vi "ConvertDMDTypeToHumanReadable.vi"(11 "UserVarPtr in":i32) -> (3 "String":string)   [LabVIEW 2013, in "alpD41.lvlib"]
uses:
  alpD41.lvlib
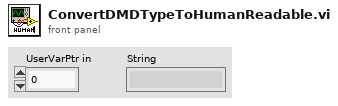
[diagram p1: front panel]
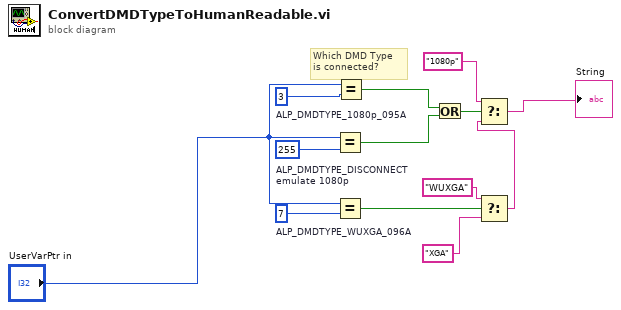
[diagram p0: block diagram]
diagram:
  w5 = u32 7  # ALP_DMDTYPE_WUXGA_096A
  w1 = u32 255  # ALP_DMDTYPE_DISCONNECT emulate 1080p
  w2 = u32 3  # ALP_DMDTYPE_1080p_095A
  # "Which DMD Type\nis connected?"
  n1 = Equal?(x="UserVarPtr in", y=w1) -> (x = y?=w4:bool)
  n2 = Equal?(x="UserVarPtr in", y=w5) -> (x = y?=w6:bool)
  n3 = Equal?(x="UserVarPtr in", y=w2) -> (x = y?=w3:bool)
  n4 = Or(x=w3, y=w4) -> (x .or. y?=w8:bool)
  n5 = Select(t="WUXGA", s=w6, f="XGA") -> (s? t:f=w10:string)
  n6 = Select(t="1080p", s=w8, f=w10) -> (s? t:f=→"String":string)
